vi "Write CS++RTMainActor.vi"(8 "Error In":errorcluster, 10 "CS++RTMainActor":refnum<class "CS++RTMainActor.lvclass">, 11 "CS++RTRootActor in":refnum<class "CS++RTRootActor.lvclass">) -> (0 "Error Out":errorcluster, 3 "CS++RTRootActor out":refnum<class "CS++RTRootActor.lvclass">)   [LabVIEW 2016, in "CS++RTRoot.lvlib" / "CS++RTRootActor.lvclass"]
doc: "Write CS++RTMainActor class to attribute."
uses:
  CS++RTRootActor.lvclass
  CS++RTMain/CS++RTMainActor.lvclass
  CS++RTRootActor.lvclass/CS++RTRootActor.ctl
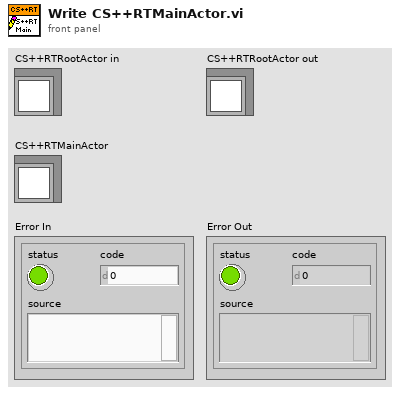
[diagram p1: front panel]
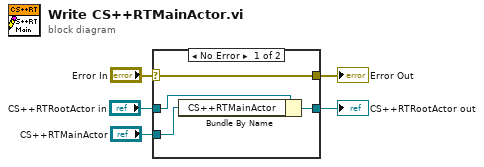
[diagram p0: block diagram]
diagram:
  n1 = case shown="No Error" "Error In" {
    selector: "Error In" -> [w9 w10]
    tunnel: [w9 w10] -> w4
    tunnel: [w7 w11] -> w2
    tunnel: "CS++RTRootActor in" -> [w8 w11]
    tunnel: "CS++RTMainActor" -> [w6 _]
    frame No Error {
      n2 = Bundle By Name(cluster=w8, "CS++RTMainActor"=w6) -> (w7:refnum<class "CS++RTRootActor.lvclass">)
    }
    frame Error {
    }
  }
  "Error Out" <- w4
  "CS++RTRootActor out" <- w2
